vi "Client Single Connection1.vi"() -> ()   [LabVIEW 2021]
doc: "Demonstrates how to use Modbus functions to create a master communicating with a Modbus slave. It shows an interactive UI to allow users manually read and write the coils on the slave using TCP connection. Users can also change the timeout for reading operation if the network state is not good."
uses:
  WebSockets/WebSocket/WebSocket.lvclass/WebSocket.ctl
  WebSockets/Timing/Calculate Timeout.vi
  WebSockets/WebSocket/Low-Level Read.vi
  WebSockets/WebSocket/Pong.vi
  WebSockets/Timing/Tick Count with Error Wires.vi
  WebSockets/WebSocket/Socket Read.vi
  WebSockets/WebSocket/Low-Level Write.vi
  WebSockets/WebSocket/DataLengthBytes.vi
  WebSockets/WebSocket/EncodeMaskedBytes.vi
  WebSockets/WebSocket/Socket Write.vi
  WebSockets/WebSocket Client/WebSocket Client.lvclass
  D:/my_projects/projects/21/WebSockets/Source/WebSockets/WebSocket/WebSocket.lvclass
  <vilib>/Utility/error.llb/Error Cluster From Error Code.vi
  WebSockets/WebSocket/DecodeMaskedBytes.vi
  Sockets/Socket/Socket.lvclass
  WebSockets/WebSocket/WebSocket.lvclass
  <vilib>/addons/Tools/Unicode/UTF8 Tools.lvlib
panel:
  in  "write period":u32=500
  out "Num of masters":u8
  in  "Data":string
  out "Chart":dbl(graph)
  out "Received Data":string
  out "HTTP Headers":variant
  in  "WebSockets URL":string="ws://echo.websocket.org"
  out "timer":u32(graph)
  in  "Stop":bool
  in  "Read":bool
  in  "Write":bool
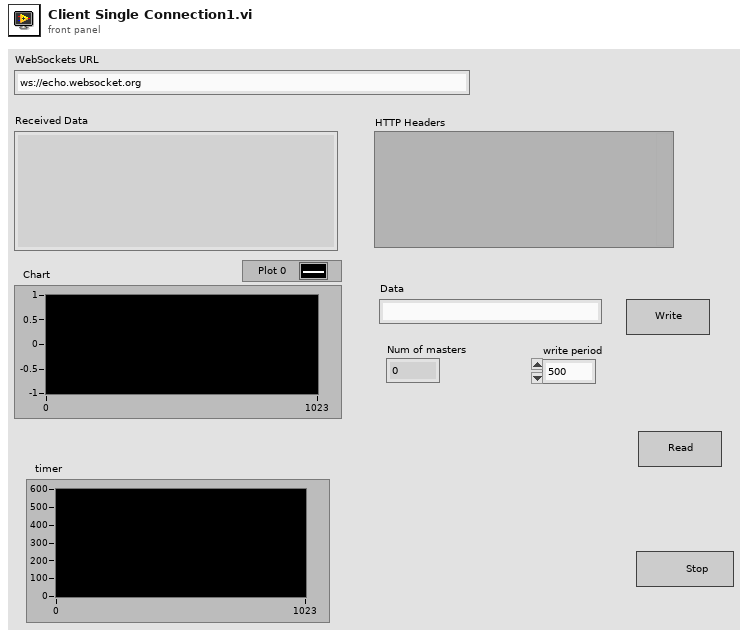
[diagram p1: front panel]
types:
  T1 = typedef "WebSockets.lvlib/WebSocket.lvclass/Opcodes.ctl" = u8
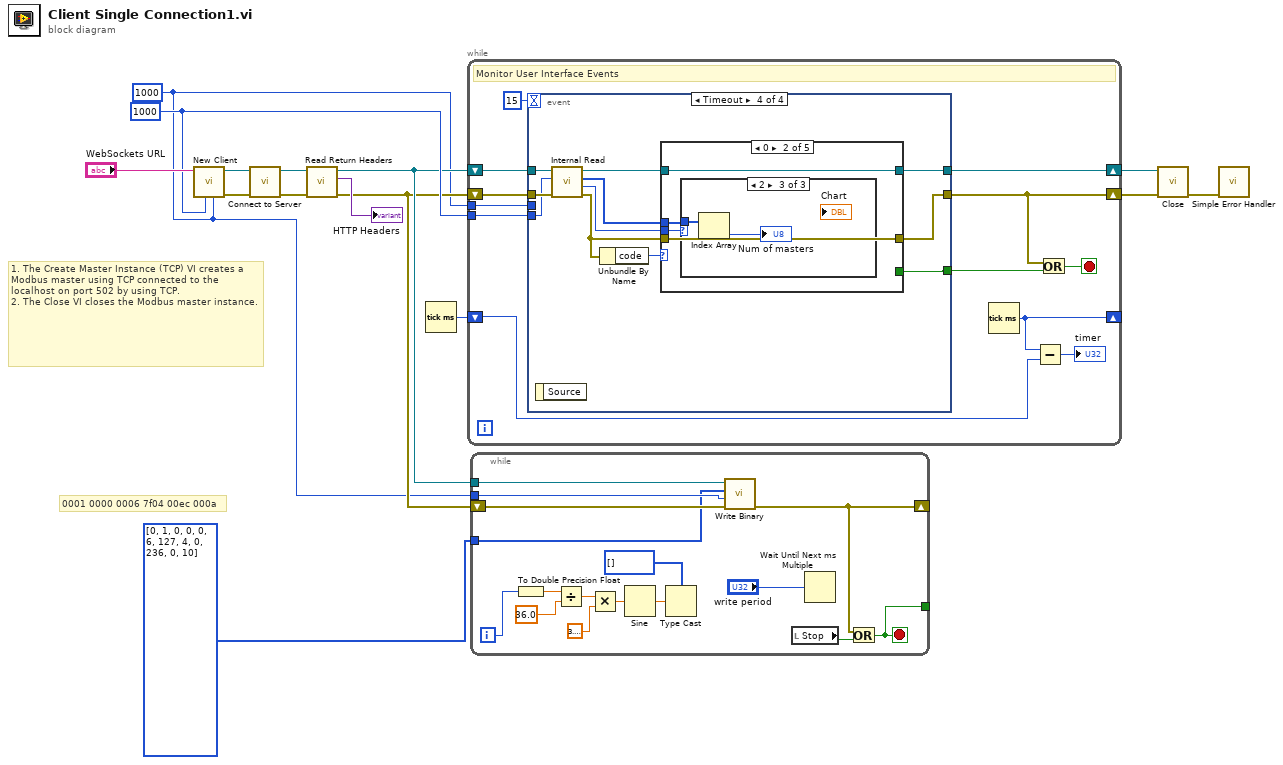
[diagram p0: block diagram]
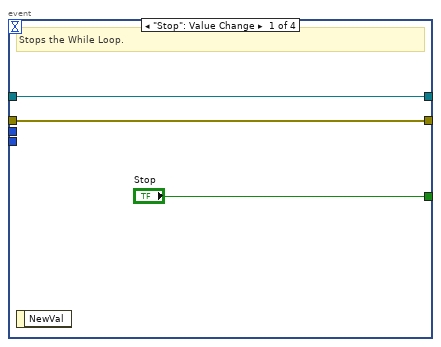
[diagram p2: hidden frame]
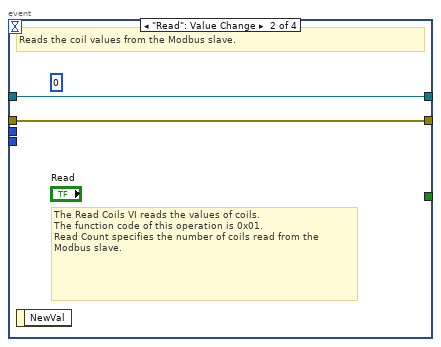
[diagram p3: hidden frame]
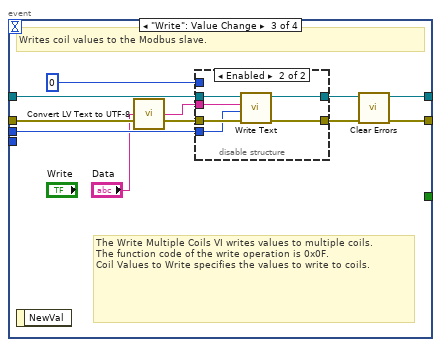
[diagram p4: hidden frame]
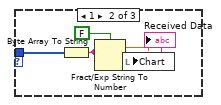
[diagram p8: hidden frame]
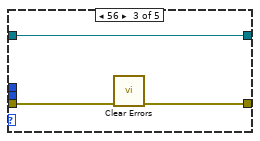
[diagram p9: hidden frame]
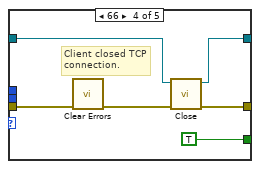
[diagram p10: hidden frame]
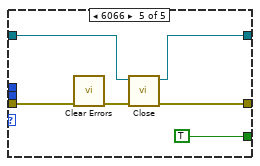
[diagram p11: hidden frame]
diagram:
  w7 = 1000 ("write operation timeout")
  w4 = 1000 ("read operation timeout")
  # "0001 0000 0006 7f04 00ec 000a"
  # "1. The Create Master Instance (TCP) VI creates a Modbus master using TCP connected to the localhost on port 502 by using TCP.\n2. The Close VI closes the Modbus master instance."
  n1 = call "New Client.vi"("write operation timeout"=w4, "read operation timeout"=w7, "WebSocket URL"="WebSockets URL") -> ("error out"=w9:errorcluster, "WebSocket Client out"=w10:refnum<class "WebSocket Client.lvclass">)  [unwired: 7 in]
  n2 = call "Connect to Server.vi"("error in (no error)"=w9, "WebSocket Client in"=w10) -> ("error out"=w2:errorcluster, "WebSocket Client out"=w3:refnum<class "WebSocket Client.lvclass">)  [unwired: 8 in]
  n3 = call "Read Return Headers.vi"("error in (no error)"=w2, "WebSocket in"=w3) -> ("error out"=w5:errorcluster, "Return Headers"=→"HTTP Headers":variant, "WebSocket out"=w6:refnum<class "WebSocket Client.lvclass">)  [unwired: 7 in]
  n4 = Tick Count (ms)() -> (millisecond timer value=w15:u32)
  n5 = while {
    shift-right: [w26] -> w13
    shift-left: w6 -> [w27]
    shift-right: [w24] -> w12
    shift-left: w5 -> [w25]
    shift-right: [w19] -> _
    shift-left: w15 -> [w20]
    tunnel: w4 -> [w17]
    tunnel: w7 -> [w16]
    stop <- w22 stop-if-true
    # "Monitor User Interface Events"
    n6 = event shown="[3] Timeout" {
      selector: _ -> [_ _ _ _]
      dyn-events: _ -> [_ _ _ _]
      timeout: 15 -> [_ _ _ _]
      tunnel: ["Stop" _ _ w55] -> w23
      tunnel: w27 -> [w29 w31 w41 w58]
      tunnel: [w29 w31 w40 w64] -> w26
      tunnel: w25 -> [w30 w32 w36 w57]
      tunnel: [w30 w32 w38 w65] -> w24
      tunnel: w17 -> [_ _ w39 _]
      tunnel: w16 -> [_ _ _ w56]
      event "Stop": Value Change {
        # "Stops the While Loop."
        n7 = event-data() -> ()  [unwired: 1 in, 1 out]
      }
      event "Read": Value Change {
        (unwired) u16 0 ("starting address")
        # "The Read Coils VI reads the values of coils.\nThe function code of this operation is 0x01.\nRead Count specifies the number of coils read from the Modbus slave."
        # "Reads the coil values from the Modbus slave."
        n8 = event-data() -> ()  [unwired: 1 in, 1 out]
      }
      event "Write": Value Change {
        # "The Write Multiple Coils VI writes values to multiple coils.\nThe function code of the write operation is 0x0F.\nCoil Values to Write specifies the values to write to coils."
        # "Writes coil values to the Modbus slave."
        n9 = event-data() -> ()  [unwired: 1 in, 1 out]
        n10 = call <vilib>:"Convert LV Text to UTF-8.vi"("LV Text"="Data", "error in"=w36) -> ("UTF-8 Text"=w33:string, "error out"=w35:errorcluster)  [unwired: 12 in]
        n11 = disable-structure shown="Enabled" {
          disable-tunnel: u16 0 ("starting address") -> [w48 _]
          disable-tunnel: w41 -> [w47 w54]
          disable-tunnel: [w46 w52] -> w40
          disable-tunnel: w35 -> [w45 w51]
          disable-tunnel: [w44 w53] -> w37
          disable-tunnel: w33 -> [w43 w50]
          disable-tunnel: w39 -> [_ w49]
          frame Disabled {
          }
          frame Enabled {
            n12 = call-dynamic "Write Text.vi"("error in (no error)"=w51, "timeout ms (5000)"=w49, "String Data"=w50, "WebSocket in"=w54) -> ("error out"=w53:errorcluster, "WebSocket out"=w52:refnum<class "WebSocket Client.lvclass">)  [unwired: 6 in]
          }
        }
        n13 = call <vilib>:"Clear Errors.vi"("error in (no error)"=w37) -> ("error out"=w38:errorcluster)  [unwired: 5 in, 1 out]
      }
      event Timeout {
        n14 = event-data() -> ()  [unwired: 1 in, 1 out]
        n15 = call "Internal Read.vi"("error in (no error)"=w57, "timeout ms"=w56, "WebSocket in"=w58) -> ("error out"=w60:errorcluster, "Opcode"=w59:T1, "Data"=w61:u8[], "WebSocket out"=w62:refnum<class "WebSocket Client.lvclass">)  [unwired: 5 in]
        n16 = Unbundle By Name(w60) -> ("code"=w63:i32)
        n17 = case shown="0" w63 {
          tunnel: w61 -> [_ w71 _ _ _]
          tunnel: [w67 w70 w79 w83 w89] -> w65
          tunnel: w60 -> [w67 w70 w80 w86 w91]
          tunnel: w62 -> [w66 w69 w78 w81 w92]
          tunnel: [w66 w69 w78 w82 w87] -> w64
          tunnel: w59 -> [_ w68 _ _ _]
          tunnel: [_ _ _ TRUE ("Stop") TRUE ("Stop")] -> w55
          frame Default {
          }
          frame 0 {
            n18 = case shown="2" w68 {
              tunnel: w71 -> [_ w75 w77]
              frame 0, Default {
              }
              frame 1 {
                n19 = Byte Array To String(unsigned byte array=w75) -> (string=w74:string)
                "Received Data" <- w74
                n20 = Fract/Exp String To Number(use system decimal point (T)=FALSE, string=w74) -> (number=w73:dbl)  [unwired: 2 in, 1 out]
                n21 = local write "Chart"(w73) -> ()
              }
              frame 2 {
                n22 = Index Array(array=w77) -> (element=→"Num of masters":u8)  [unwired: 1 in]
              }
            }
          }
          frame 56 {
            n23 = call <vilib>:"Clear Errors.vi"("error in (no error)"=w80) -> ("error out"=w79:errorcluster)  [unwired: 5 in, 1 out]
          }
          frame 66 {
            # "Client closed TCP connection."
            n24 = call <vilib>:"Clear Errors.vi"("error in (no error)"=w86) -> ("error out"=w84:errorcluster)  [unwired: 5 in, 1 out]
            n25 = call-dynamic "Close.vi"("error in (no error)"=w84, "WebSocket Client in"=w81) -> ("error out"=w83:errorcluster, "WebSocket Client out"=w82:refnum<class "WebSocket Client.lvclass">)  [unwired: 8 in]
          }
          frame 6066 {
            n26 = call <vilib>:"Clear Errors.vi"("error in (no error)"=w91) -> ("error out"=w90:errorcluster)  [unwired: 5 in, 1 out]
            n27 = call-dynamic "Close.vi"("error in (no error)"=w90, "WebSocket Client in"=w92) -> ("error out"=w89:errorcluster, "WebSocket Client out"=w87:refnum<class "WebSocket Client.lvclass">)  [unwired: 8 in]
          }
        }
      }
    }
    n28 = Tick Count (ms)() -> (millisecond timer value=w19:u32)
    n29 = Subtract(x=w19, y=w20) -> (x-y=→"timer":u32)
    n30 = Or(x=w24, y=w23) -> (x .or. y?=w22:bool)
  }
  n31 = while {
    tunnel: w6 -> [w97]
    tunnel: [w107] -> _
    shift-right: [w96] -> _
    shift-left: w5 -> [w95]
    tunnel: w4 -> [w94]
    tunnel: u8[] [0, 1, 0, 0, 0, 6, 127, 4, 0, 236, 0, 10] ("values") -> [w93]
    i -> [w98]
    stop <- w107 stop-if-true
    n32 = To Double Precision Float(number=w98) -> (double precision float=w105:dbl)
    n33 = Divide(x=w105, y=36.0) -> (x/y=w104:dbl)
    n34 = Multiply(x=w104, y=3.141592653589793) -> (x*y=w103:dbl)
    n35 = Sine(x=w103) -> (sin(x)=w102:dbl)
    n36 = Type Cast(type=u8[] [] ("values"), x=w102) -> ()  [unwired: 1 out]
    n37 = call-dynamic "Write Binary.vi"("error in (no error)"=w95, "timeout ms (5000)"=w94, "Binary Data"=w93, "WebSocket in"=w97) -> ("error out"=w96:errorcluster)  [unwired: 6 in, 1 out]
    n38 = local read "Stop"() -> (w108:bool)
    n39 = Wait Until Next ms Multiple(millisecond multiple="write period") -> ()  [unwired: 1 out]
    n40 = Or(x=w96, y=w108) -> (x .or. y?=w107:bool)
  }
  n41 = call-dynamic "Close.vi"("error in (no error)"=w12, "WebSocket Client in"=w13) -> ("error out"=w11:errorcluster)  [unwired: 8 in, 1 out]
  n42 = call <vilib>:"Simple Error Handler.vi"("error in (no error)"=w11) -> ()  [unwired: 4 in, 5 out]
